vi "Ini_SetOutput.vi"(8 "error in (no error)":errorcluster, 11 "6480 in":refnum<class "6480.lvclass">) -> (0 "error out":errorcluster, 3 "6480 out":refnum<class "6480.lvclass">)   [LabVIEW 2019, in "6480.lvclass"]
uses:
  6480.lvclass
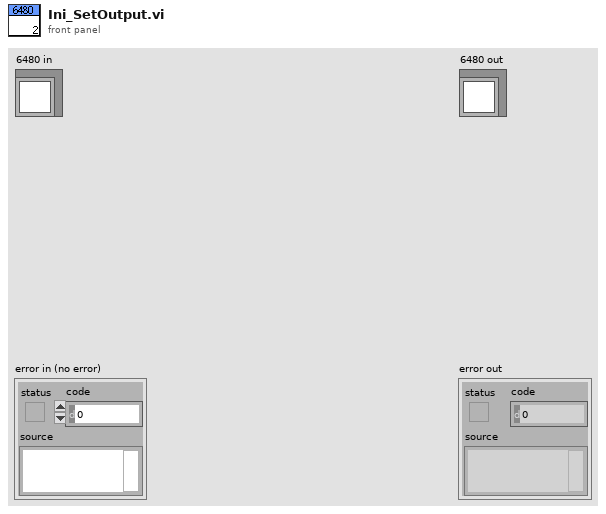
[diagram p1: front panel]
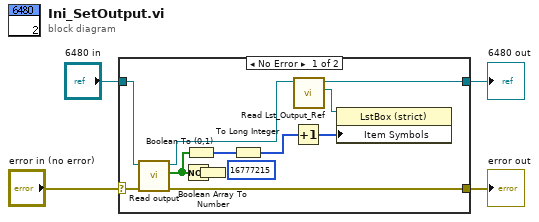
[diagram p0: block diagram]
diagram:
  n1 = case shown="No Error" "error in (no error)" {
    selector: "error in (no error)" -> [w15 w16]
    tunnel: "6480 in" -> [w14 w17]
    tunnel: [w5 w16] -> w2
    tunnel: [w8 w17] -> w1
    frame No Error {
      (unwired) u32 16777215 ("port_value")
      n2 = call-dynamic "Read output.vi"("error in (no error)"=w15, "IOCard in"=w14) -> ("error out"=w5:errorcluster, "output"=w7:bool[], "IOCard out"=w9:refnum<class "6480.lvclass">)  [unwired: 7 in]
      n3 = Not(x=w7) -> (.not. x?=w6:bool[])
      n4 = Boolean To (0,1)(Boolean=w7) -> (0, 1=w12:i16[])
      n5 = Boolean Array To Number(Boolean array=w6) -> ()  [unwired: 1 out]
      n6 = To Long Integer(number=w12) -> (32bit integer=w11:i32[])
      n7 = Increment(x=w11) -> (x+1=w10:i32[])
      n8 = call-dynamic "Read Lst_Output_Ref.vi"("IOCard in"=w9) -> ("Lst_Output_Ref"=w13:refnum<vi>, "IOCard out"=w8:refnum<class "6480.lvclass">)  [unwired: 8 in, 1 out]
      n9 = property class="LstBox (strict)"(reference=w13, "Item Symbols"=w10) -> ()  [unwired: 1 in, 2 out]
    }
    frame Error {
    }
  }
  "error out" <- w2
  "6480 out" <- w1
